vi "robotprofile.vi"() -> ()   [LabVIEW 2019]
doc: "This global variable contains information that allows similar, but not identical, robots (e.g. an Alpha and a Beta) run identical code bases."
panel:
  out "Pressure_Transducer_Bypass":bool
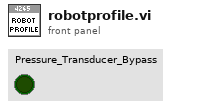
[diagram p1: front panel]
diagram:
